vi "main - Client.vi"() -> ()   [LabVIEW 2024]
uses:
  <vilib>/Instr/_visa.llb/VISA Configure Serial Port (Instr).vi
panel:
  in  "Clr?":bool
  out "Iterations":i32=266
  in  "Tx":bool
  in  "Tx String":string
  in  "Serial Port":refnum<visa-resource-name>="COM4"
  in  "Clear":bool
  out "error out":errorcluster={"status"=FALSE, "code"=1073676294, "source"="VISA Read in main - Client.vi"}
  in  "Stop":bool
  out "Console":string="I (24751) BLE_INIT: BT controller compile version [d752dea]\r\nI (24751) BLE_INIT: Bluetooth MAC: 34:cd:b0:0a:1f:7a\r\nI (24751) phy_init: phy_version 680,a6008b2,Jun  4 2024,16:41:10\r\nI (24791) GATTC_SPP_DEMO: app_main init bluetooth\r\nI (24811) GATTC_SPP_DEMO: register callback\r\nI (24811) GATTC_SPP_DEMO: EVT 0, gattc if 3\r\nI (24811) GATTC_SPP_DEMO: gattc_profile_event_handler():\r\n  //----------------------------------------------------------------------------------------------------//\r\nI (24821) GATTC_SPP_DEMO: REG EVT, set scan params\r\nI (24821) GATTC_SPP_DEMO: Enable Ble Scan:during time ffff minutes.\r\nI (24831) GATTC_SPP_DEMO: Scan start successfully\r\nI (24831) uart: queue free spaces: 10\r\nI (24831) GATTC_SPP_DEMO: 48 e7 29 a3 b6 52\r\nI (24841) GATTC_SPP_DEMO: Searched Adv Data Len 23, Scan Response Len 0\r\nI (24851) GATTC_SPP_DEMO: Searched Device Name Len 14\r\nI (24851) GATTC_SPP_DEMO: ESP_SPP_SERVER\r\nI (24851) GATTC_SPP_DEMO:  \r\nI (24861) GATTC_SPP_DEMO: Scan stop successfully\r\nI (24861) GATTC_SPP_DEMO: Connect to the remote device.\r\nI (24871) main_task: Returned from app_main()\r\nI (24951) GATTC_SPP_DEMO: EVT 40, gattc if 3\r\nI (24951) GATTC_SPP_DEMO: gattc_profile_event_handler():\r\n  //----------------------------------------------------------------------------------------------------//\r\nI (24961) GATTC_SPP_DEMO: ESP_GATTC_CONNECT_EVT: conn_id=0, gatt_if = 3\r\nI (24961) GATTC_SPP_DEMO: REMOTE BDA:\r\nI (24971) GATTC_SPP_DEMO: 00 00 00 00 00 00\r\nI (24971) GATTC_SPP_DEMO: EVT 2, gattc if 3\r\nI (24981) GATTC_SPP_DEMO: gattc_profile_event_handler():\r\n  //----------------------------------------------------------------------------------------------------//\r\nI (25801) GATTC_SPP_DEMO: EVT 46, gattc if 3\r\nI (25801) GATTC_SPP_DEMO: gattc_profile_event_handler():\r\n  //----------------------------------------------------------------------------------------------------//\r\nI (25811) GATTC_SPP_DEMO: EVT 7, gattc if 3\r\nI (25811) GATTC_SPP_DEMO: gattc_profile_event_handler():\r\n  //----------------------------------------------------------------------------------------------------//\r\nI (25831) GATTC_SPP_DEMO: ESP_GATTC_SEARCH_RES_EVT: start_handle = 40, end_handle = 65535, UUID:0xabf0\r\nI (25831) GATTC_SPP_DEMO: EVT 6, gattc if 3\r\nI (25841) GATTC_SPP_DEMO: gattc_profile_event_handler():\r\n  //----------------------------------------------------------------------------------------------------//\r\nI (25851) GATTC_SPP_DEMO: SEARCH_CMPL: conn_id = 0, status 0\r\nI (25901) GATTC_SPP_DEMO: EVT 18, gattc if 3\r\nI (25901) GATTC_SPP_DEMO: gattc_profile_event_handler():\r\n  //----------------------------------------------------------------------------------------------------//\r\nI (25911) GATTC_SPP_DEMO: +MTU:200\r\nI (25911) GATTC_SPP_DEMO: attr_type = PRIMARY_SERVICE,attribute_handle=40,start_handle=40,end_handle=65535,properties=0x0,uuid=0xabf0\r\nI (25921) GATTC_SPP_DEMO: attr_type = CHARACTERISTIC,attribute_handle=42,start_handle=0,end_handle=0,properties=0x6,uuid=0xabf1\r\nI (25931) GATTC_SPP_DEMO: attr_type = CHARACTERISTIC,attribute_handle=44,start_handle=0,end_handle=0,properties=0x12,uuid=0xabf2\r\nI (25941) GATTC_SPP_DEMO: attr_type = DESCRIPTOR,attribute_handle=45,start_handle=0,end_handle=0,properties=0x0,uuid=0x2902\r\nI (25951) GATTC_SPP_DEMO: attr_type = CHARACTERISTIC,attribute_handle=47,start_handle=0,end_handle=0,properties=0x6,uuid=0xabf3\r\nI (25961) GATTC_SPP_DEMO: attr_type = CHARACTERISTIC,attribute_handle=49,start_handle=0,end_handle=0,properties=0x12,uuid=0xabf4\r\nI (25981) GATTC_SPP_DEMO: attr_type = DESCRIPTOR,attribute_handle=50,start_handle=0,end_handle=0,properties=0x0,uuid=0x2902\r\nI (25991) GATTC_SPP_DEMO: Index = 2,UUID = 0xabf2, handle = 44\r\nI (25991) GATTC_SPP_DEMO: EVT 38, gattc if 3\r\nI (26001) GATTC_SPP_DEMO: gattc_profile_event_handler():\r\n  //----------------------------------------------------------------------------------------------------//\r\nI (26011) GATTC_SPP_DEMO: Index = 2,status = 0, handle = 44\r\nI (26051) GATTC_SPP_DEMO: EVT 9, gattc if 3\r\nI (26051) GATTC_SPP_DEMO: gattc_profile_event_handler():\r\n  //----------------------------------------------------------------------------------------------------//\r\nI (26061) GATTC_SPP_DEMO: ESP_GATTC_WRITE_DESCR_EVT: status = 0, handle = 45\r\nI (26091) GATTC_SPP_DEMO: Index = 5,UUID = 0xabf4, handle = 49\r\nI (26091) GATTC_SPP_DEMO: EVT 38, gattc if 3\r\nI (26091) GATTC_SPP_DEMO: gattc_profile_event_handler():\r\n  //----------------------------------------------------------------------------------------------------//\r\nI (26101) GATTC_SPP_DEMO: Index = 5,status = 0, handle = 49\r\nI (26151) GATTC_SPP_DEMO: EVT 9, gattc if 3\r\nI (26151) GATTC_SPP_DEMO: gattc_profile_event_handler():\r\n  //----------------------------------------------------------------------------------------------------//\r\nI (26161) GATTC_SPP_DEMO: ESP_GATTC_WRITE_DESCR_EVT: status = 0, handle = 50\r\n"
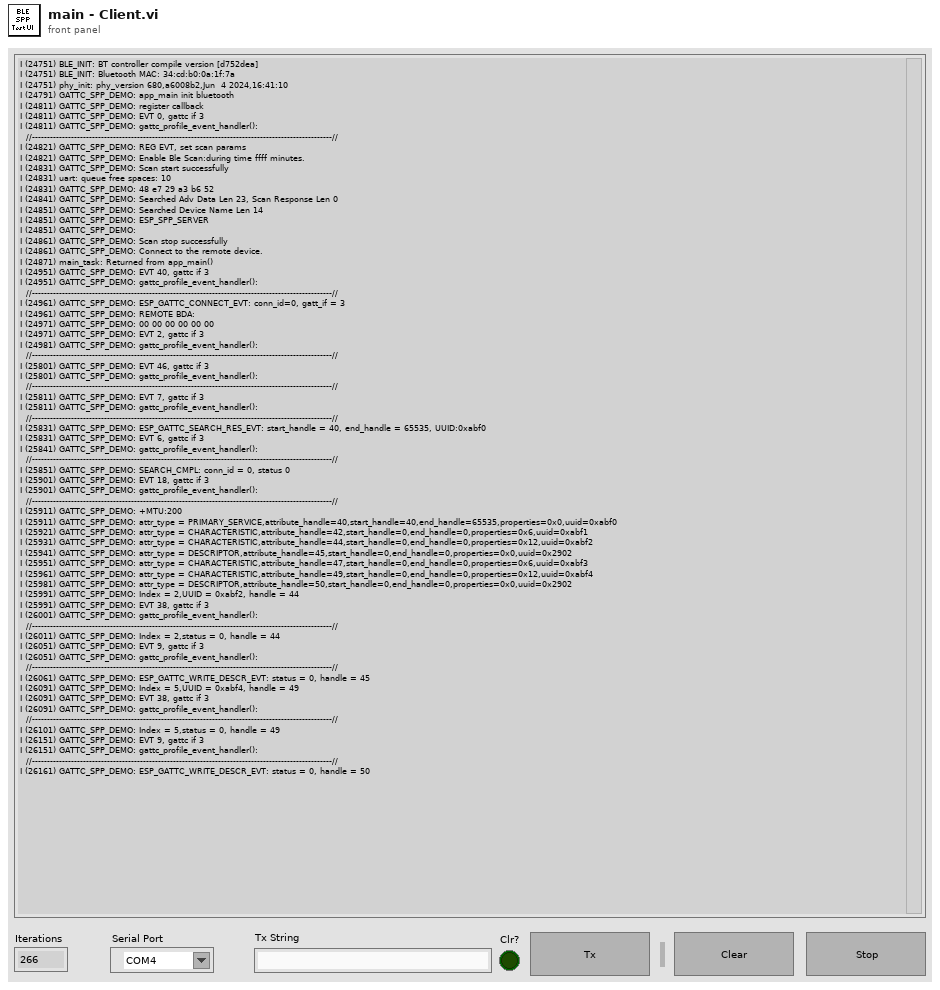
[diagram p1: front panel]
types:
  T1 = enum8{"Enabled", "Disabled", "Disabled and Grayed Out"}
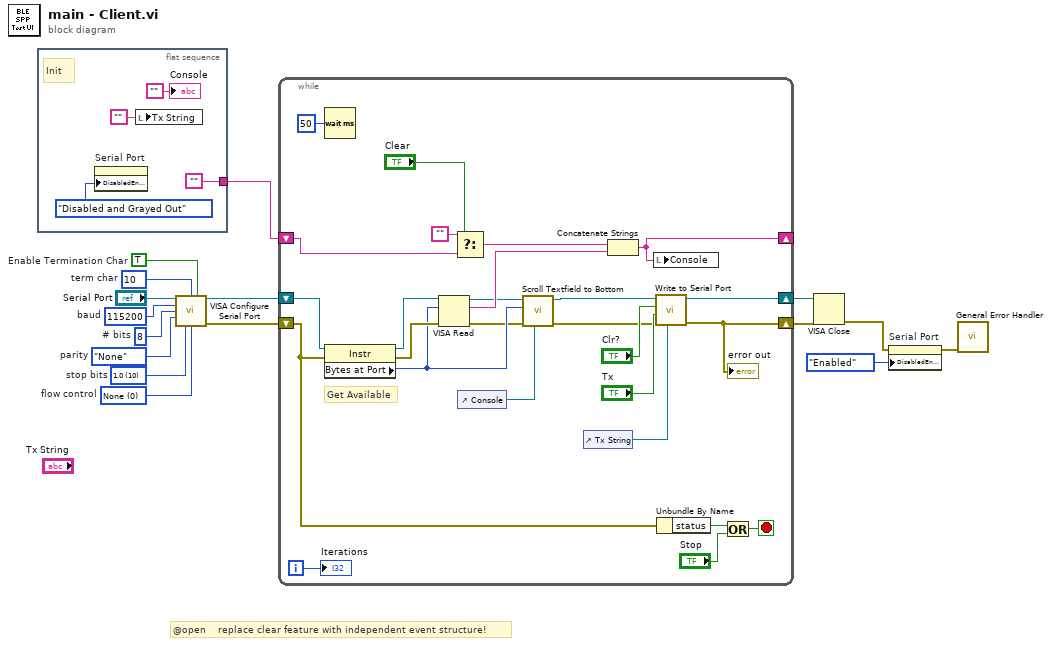
[diagram p0: block diagram]
diagram:
  w10 = u8 10  # term char
  w11 = u16 0 items=["None", "XON/XOFF", "RTS/CTS", "XON/XOFF & RTS/CTS", "DTR/DSR", "XON/XOFF & DTR/DSR"]  # flow control
  w12 = TRUE  # Enable Termination Char
  w13 = u16 10 items=["1.0"=10, "1.5"=15, "2.0"=20]  # stop bits
  w14 = enum16{"None", "Odd", "Even", "Mark", "Space"}."None"  # parity
  w15 = u16 8  # # bits
  w16 = u32 115200  # baud
  # "@open    replace clear feature with independent event structure!"
  n1 = flat-sequence {
    tunnel: [""] -> w4
    frame #0 {
      # "Init"
      n2 = property on="Serial Port" class="VISAName"("DisabledEnum"=T1."Disabled and Grayed Out" ("Disabled")) -> ()  [unwired: 2 in, 2 out]
      n3 = local write "Tx String"("") -> ()
      "Console" <- ""
    }
  }
  n4 = call-poly "VISA Configure Serial Port"("VISA resource name"="Serial Port", "termination char\n(0xA = '\\n' = LF)"=w10, "Enable Termination\nChar (T)"=w12, "baud rate (9600)"=w16, "data bits (8)"=w15, "parity (0:none)"=w14, "stop bits (10: 1 bit)"=w13, "flow control (0:none)"=w11) -> ("VISA resource name out"=w9:refnum<visa-resource-name>, "error out"=w8:errorcluster)  [unwired: 6 in]
  n5 = while {
    shift-right: [w29] -> w6
    shift-left: w9 -> [w38]
    shift-right: [w31] -> w7
    shift-left: w8 -> [w35]
    shift-right: [w39] -> _
    shift-left: w4 -> [w42]
    i -> [w26]
    stop <- w44 stop-if-true
    # "Get Available"
    n6 = Wait (ms)(milliseconds to wait=u32 50) -> ()  [unwired: 1 out]
    n7 = property class="Instr"(reference=w38, error in=w35) -> (reference out=w37:refnum<visa-resource-name>, error out=w36:errorcluster, "Bytes at Port"=w33:u32)
    n8 = VISA Read(VISA resource name=w37, byte count=w33, error in (no error)=w36) -> (VISA resource name out=w22:refnum<visa-resource-name>, read buffer=w41:string, error out=w32:errorcluster)  [unwired: 1 out]
    n9 = Select(t="", s="Clear", f=w42) -> (s? t:f=w40:string)
    n10 = control-ref of="Console"() -> (w28:refnum<vi>)
    n11 = call "Scroll Textfield to Bottom.vi"("Console String"=w28, "error in (no error)"=w32, "Bytes at Serial Port"=w33, "VISA refnum in"=w22) -> ("error out"=w24:errorcluster, "VISA refnum out"=w23:refnum<visa-resource-name>)  [unwired: 6 in]
    n12 = control-ref of="Tx String"() -> (w27:refnum<vi>)
    n13 = Concatenate Strings(w40, w41) -> (w39:string)
    n14 = local write "Console"(w39) -> ()
    n15 = call "Write to Serial Port.vi"("Tx String"=w27, "error in (no error)"=w24, "Transmit?"="Tx", "Clear after send?"="Clr?", "VISA refnum in"=w23) -> ("error out"=w31:errorcluster, "VISA refnum out"=w29:refnum<visa-resource-name>)  [unwired: 5 in]
    "error out" <- w31
    n16 = Unbundle By Name(w35) -> ("status"=w46:bool)
    n17 = Or(x=w46, y="Stop") -> (x .or. y?=w44:bool)
    "Iterations" <- w26
  }
  n18 = VISA Close(VISA resource name=w6, error in (no error)=w7) -> (error out=w2:errorcluster)
  n19 = property on="Serial Port" class="VISAName"(error in=w2, "DisabledEnum"=T1."Enabled" ("Disabled")) -> (error out=w3:errorcluster)  [unwired: 1 in, 1 out]
  n20 = call <vilib>:"General Error Handler.vi"("error in (no error)"=w3) -> ()  [unwired: 10 in, 5 out]
